vi "Fgen Sweep Generator.vi"() -> ()   [LabVIEW 2021]
doc: "This example shows how to use the Frequency List mode to generate a frequency sweep."
uses:
  <instrlib>/niFgen/niFgen.llb/niFgen Output Mode.ctl
  <instrlib>/niFgen/niFgen.llb/niFgen Disable Start Trigger.vi
  <instrlib>/niFgen/niFgen.llb/niFgen Configure Software Edge Start Trigger.vi
  <instrlib>/niFgen/niFgen.llb/niFgen Configure Digital Edge Start Trigger.vi
panel:
  out "Done":bool
  in  "Stop":bool
  in  "Waveform":u16(ring) items=["Sine", "Square", "Triangle", "Ramp Up", "Ramp Down", "DC", "Noise"]
  in  "Trigger Source":string(combo)="PFI0"
  in  "Trigger Mode":u16(ring)=1 items=["Single", "Continuous", "Stepped", "Burst"]
  in  "Trigger Type":u16(ring) items=["None", "Software Edge", "Digital Edge"]
  in  "Stop Frequency":dbl=1000000.0 format="%.2p"
  in  "Duration (s) / Step":dbl=0.01 format="%.2p"
  in  "DC Offset":dbl format="%.2f"
  in  "Amplitude":dbl=2.0 format="%.2f"
  in  "# of Frequency Steps":i32=512
  in  "Start Frequency":dbl=1000.0 format="%.2p"
  in  "FGEN Resource Name":refnum<k15>
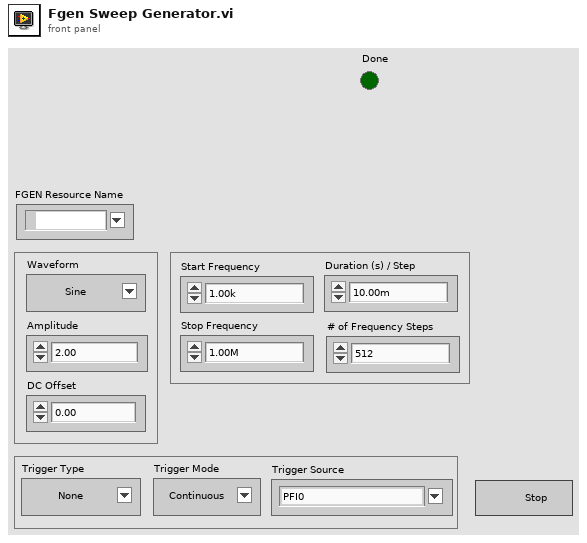
[diagram p1: front panel]
types:
  T1 = typedef "niFgen Output Mode.ctl" = u32
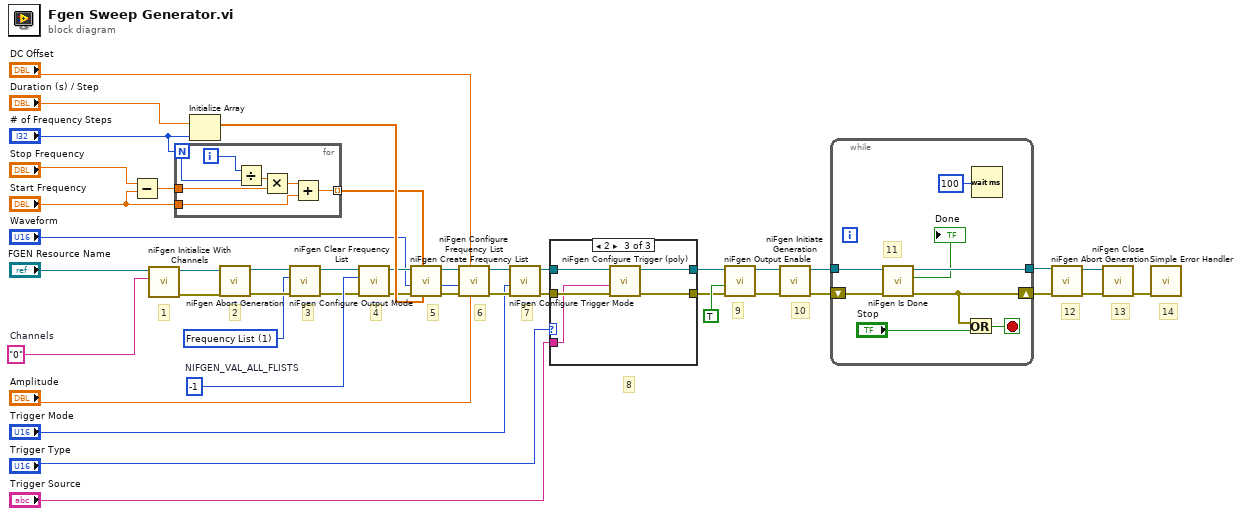
[diagram p0: block diagram]
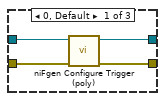
[diagram p2: hidden frame]
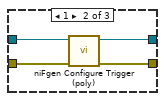
[diagram p3: hidden frame]
diagram:
  w4 = "0"  # Channels
  w6 = T1 1 items=["Standard Function", "Frequency List", "Arbitrary Waveform", "Arbitrary Sequence", "Script"] ("output mode")
  w37 = -1  # NIFGEN_VAL_ALL_FLISTS
  # "14"
  # "13"
  # "12"
  # "10"
  # "9"
  # "8"
  # "7"
  # "6"
  # "5"
  # "4"
  # "3"
  # "2"
  # "1"
  n1 = Subtract(x="Stop Frequency", y="Start Frequency") -> (x-y=w25:dbl)
  n2 = call <instrlib>:"niFgen Initialize With Channels.vi"("Channel Name"=w4, "Resource Name"="FGEN Resource Name") -> ("error out"=w2:errorcluster, "Instrument Handle Out"=w1:refnum<k15>)  [unwired: 8 in]
  n3 = for {
    N: "# of Frequency Steps" -> [w48]
    tunnel: [w51] -> w26 mode=indexing
    tunnel: w25 -> [w47]
    tunnel: "Start Frequency" -> [w49]
    i -> [w45]
    n4 = Divide(x=w45, y=w48) -> (x/y=w46:dbl)
    n5 = Multiply(x=w46, y=w47) -> (x*y=w50:dbl)
    n6 = Add(x=w50, y=w49) -> (x+y=w51:dbl)
  }
  n7 = Initialize Array("Duration (s) / Step", "# of Frequency Steps") -> (w44:dbl[])
  n8 = call <instrlib>:"niFgen Abort Generation.vi"("error in (no error)"=w2, "Instrument Handle"=w1) -> ("error out"=w35:errorcluster, "Instrument Handle Out"=w36:refnum<k15>)  [unwired: 8 in]
  n9 = call <instrlib>:"niFgen Configure Output Mode.vi"("error in (no error)"=w35, "Output Mode (default: 0=Standard Function)"=w6, "Instrument Handle"=w36) -> ("error out"=w33:errorcluster, "Instrument Handle Out"=w34:refnum<k15>)  [unwired: 6 in]
  n10 = call <instrlib>:"niFgen Clear Frequency List.vi"("error in (no error)"=w33, "Frequency List Handle"=w37, "Instrument Handle"=w34) -> ("error out"=w38:errorcluster, "Instrument Handle Out"=w43:refnum<k15>)  [unwired: 7 in]
  n11 = call <instrlib>:"niFgen Create Frequency List.vi"("Duration Array"=w44, "Frequency Array"=w26, "error in (no error)"=w38, "Waveform"="Waveform", "Instrument Handle"=w43) -> ("error out"=w39:errorcluster, "Frequency List Handle"=w32:i32, "Instrument Handle Out"=w42:refnum<k15>)  [unwired: 4 in]
  n12 = call <instrlib>:"niFgen Configure Frequency List.vi"("Amplitude"="Amplitude", "DC Offset"="DC Offset", "error in (no error)"=w39, "Frequency List Handle"=w32, "Instrument Handle"=w42) -> ("error out"=w28:errorcluster, "Instrument Handle Out"=w30:refnum<k15>)  [unwired: 5 in]
  n13 = call <instrlib>:"niFgen Configure Trigger Mode.vi"("error in (no error)"=w28, "Trigger Mode (default: 1=continuous)"="Trigger Mode", "Instrument Handle"=w30) -> ("error out"=w27:errorcluster, "Instrument Handle Out"=w29:refnum<k15>)  [unwired: 7 in]
  n14 = case shown="2" "Trigger Type" {
    tunnel: w29 -> [w55 w59 w64]
    tunnel: w27 -> [w54 w58 w63]
    tunnel: [w53 w57 w62] -> w24
    tunnel: [w52 w56 w61] -> w23
    tunnel: "Trigger Source" -> [_ _ w60]
    frame 0, Default {
      n15 = call-poly <instrlib>:"niFgen Configure Trigger (poly).vi"("error in (no error)"=w54, "Instrument Handle"=w55) -> ("error out"=w53:errorcluster, "Instrument Handle Out"=w52:refnum<k15>)  [unwired: 8 in]
    }
    frame 1 {
      n16 = call-poly <instrlib>:"niFgen Configure Trigger (poly).vi"("error in (no error)"=w58, "Instrument Handle"=w59) -> ("error out"=w57:errorcluster, "Instrument Handle Out"=w56:refnum<k15>)  [unwired: 8 in]
    }
    frame 2 {
      n17 = call-poly <instrlib>:"niFgen Configure Trigger (poly).vi"("error in (no error)"=w63, "Source"=w60, "Instrument Handle"=w64) -> ("error out"=w62:errorcluster, "Instrument Handle Out"=w61:refnum<k15>)  [unwired: 7 in]
    }
  }
  n18 = call <instrlib>:"niFgen Output Enable.vi"("error in (no error)"=w24, "Output Enable (default: True)"=TRUE ("output enable"), "Instrument Handle"=w23) -> ("error out"=w40:errorcluster, "Instrument Handle Out"=w41:refnum<k15>)  [unwired: 7 in]
  n19 = call <instrlib>:"niFgen Initiate Generation.vi"("error in (no error)"=w40, "Instrument Handle"=w41) -> ("error out"=w20:errorcluster, "Instrument Handle Out"=w19:refnum<k15>)  [unwired: 8 in]
  n20 = while {
    tunnel: w19 -> [w67]
    tunnel: [w66] -> w21
    shift-right: [w68] -> w22
    shift-left: w20 -> [w69]
    stop <- w71 stop-if-true
    # "11"
    n21 = call <instrlib>:"niFgen Is Done.vi"("error in (no error)"=w69, "Instrument Handle"=w67) -> ("error out"=w68:errorcluster, "Done"=→"Done":bool, "Instrument Handle Out"=w66:refnum<k15>)  [unwired: 7 in]
    n22 = Or(x=w68, y="Stop") -> (x .or. y?=w71:bool)
    n23 = Wait (ms)(milliseconds to wait=u32 100 ("millisecond multiple")) -> ()  [unwired: 1 out]
  }
  n24 = call <instrlib>:"niFgen Abort Generation.vi"("error in (no error)"=w22, "Instrument Handle"=w21) -> ("error out"=w17:errorcluster, "Instrument Handle Out"=w18:refnum<k15>)  [unwired: 8 in]
  n25 = call <instrlib>:"niFgen Close.vi"("error in (no error)"=w17, "Instrument Handle"=w18) -> ("error out"=w8:errorcluster)  [unwired: 9 in]
  n26 = call <vilib>:"Simple Error Handler.vi"("error in (no error)"=w8) -> ()  [unwired: 4 in, 5 out]
